vi "Write shift registers.vi"(5 "shift registers":refnum<class "ShiftRegister.lvclass">[](array[class]), 9 "Loop in":refnum<class "Loop.lvclass">) -> (3 "Loop out":refnum<class "Loop.lvclass">)   [LabVIEW 2014, in "Raspberry Pi Compatible Compiler for LabVIEW.lvlib" / "Loop.lvclass"]
uses:
  Loop.lvclass
  ShiftRegister/ShiftRegister.lvclass
  Loop.lvclass/Loop.ctl
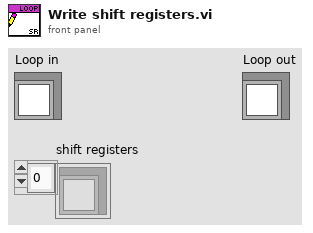
[diagram p1: front panel]
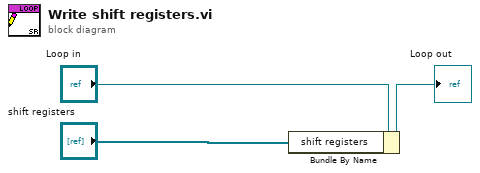
[diagram p0: block diagram]
diagram:
  n1 = Bundle By Name(cluster="Loop in", "shift registers"="shift registers") -> (→"Loop out":refnum<class "Loop.lvclass">)
